vi "ReadStimulus.vi"(8 "error in (no error)":errorcluster, 11 "StimulusObject in":refnum<class "StimulusObject.lvclass">) -> (0 "error out":errorcluster, 2 "StimulusOut":sgl[][](array[numeric]), 3 "StimulusObject out":refnum<class "StimulusObject.lvclass">)   [LabVIEW 2019, in "StimulusObject.lvclass"]
uses:
  StimulusObject.lvclass
  StimulusObject.lvclass/StimulusObject.ctl
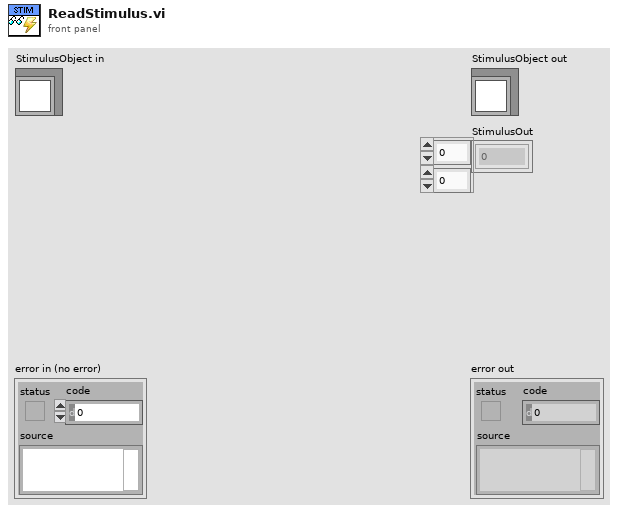
[diagram p1: front panel]
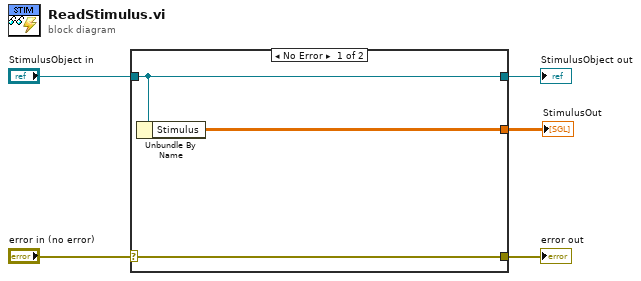
[diagram p0: block diagram]
diagram:
  n1 = case shown="No Error" "error in (no error)" {
    selector: "error in (no error)" -> [w8 w9]
    tunnel: [w8 w9] -> w4
    tunnel: [w7 w10] -> w2
    tunnel: "StimulusObject in" -> [w7 w10]
    tunnel: [w6 _] -> w1
    frame No Error {
      n2 = Unbundle By Name(w7) -> ("Stimulus"=w6:sgl[][])
    }
    frame Error {
    }
  }
  "error out" <- w4
  "StimulusObject out" <- w2
  "StimulusOut" <- w1
